vi "GUI.TestOPCConnection.vi"(8 "error in":errorcluster, 11 "Node Ptr":T1=18446744073709551615 format="%.0x") -> (0 "error out":errorcluster)   [LabVIEW 2019, in "OPC UA Client Addon System Explorer.lvlib"]
uses:
  OPC UA Client Addon System Explorer.lvlib
  <vilib>/NI VeriStand/Custom Device API/Custom Device Item Ref.ctl
  Addon Shared/SubVIs/Constants.vi
  <vilib>/NI VeriStand/Custom Device API/NI VeriStand - Get Item Property.vi
  <vilib>/NI VeriStand/Custom Device API/Get Item Property (String).vi
  <vilib>/NI VeriStand/Custom Device API/Get Item Property (U16).vi
  <vilib>/NI VeriStand/Custom Device API/Get Item Property (Dependent File).vi
  <vilib>/NI VeriStand/Custom Device API/NI VeriStand - Set Item Property.vi
  <vilib>/NI VeriStand/Custom Device API/Set Item Property (String).vi
  <vilib>/NI VeriStand/Custom Device API/Set Item Property (U16).vi
  <vilib>/Utility/libraryn.llb/Get File Extension.vi
  <vilib>/Utility/MD5Checksum.llb/MD5Checksum File.vi
  <vilib>/NI VeriStand/Custom Device API/Set Item Property (Dependent File).vi
  <vilib>/Utility/libraryn.llb/Check if File or Folder Exists.vi
  <vilib>/NI VeriStand/Custom Device API/NI VeriStand - Remove Item Property.vi
  <vilib>/OPCUA/NI OPC UA Client.lvlib
  Addon Shared/OPC UA Client Addon Shared.lvlib
  <vilib>/NI VeriStand/Custom Device API/Custom Device API.lvlib
panel:
  out "?":string="Testing..."
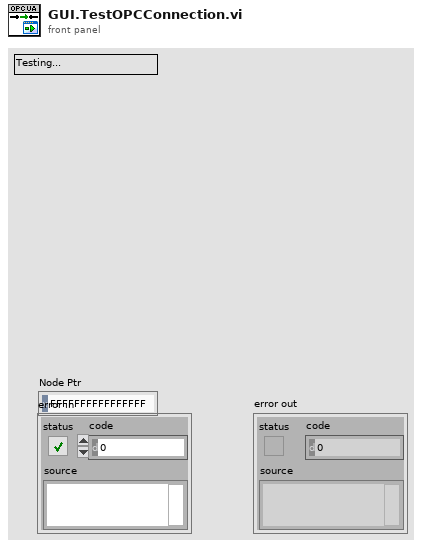
[diagram p1: front panel]
types:
  T1 = typedef "Custom Device API.lvlib/Custom Device Item Ref.ctl" = u64
  T2 = typedef "OPC UA Client Addon Shared.lvlib/OPCConnection.Properties.ctl" = cluster{"Server IP Address":string, "Server Port":u16, "Message Mode":enum16{"None", "Sign", "Sign and Encrypt"}, "Security":enum16{"Basic256", "Basic128Rsa15"}, "User Name":string, "Password":string, "Client Certificate":path, "Server Certificate":path, "Server Certificate (RT)":path, "Client Certificate (RT)":path}
  T3 = cluster{"Message Mode":enum16{"None", "Sign", "Sign and Encrypt"}, "Security":enum16{"Basic256", "Basic128Rsa15"}}
  T4 = typedef "OPC UA Client Refnum.ctl" = refnum<k21>
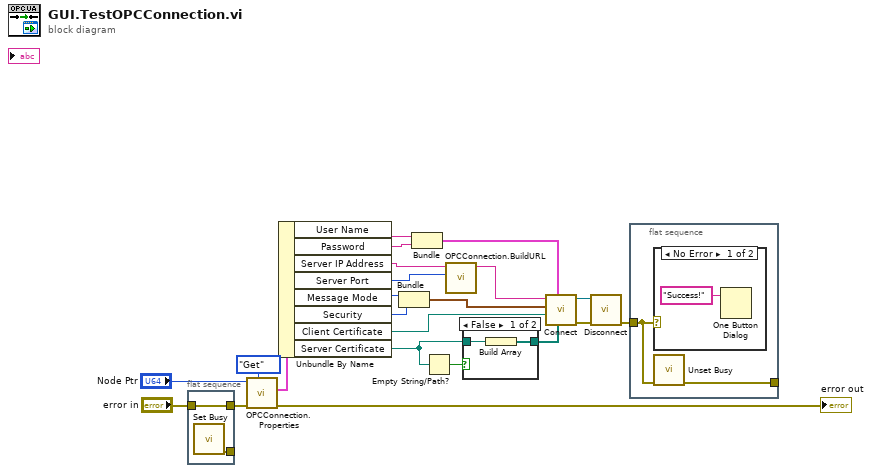
[diagram p0: block diagram]
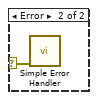
[diagram p3: hidden frame]
diagram:
  n1 = flat-sequence {
    tunnel: [w24] -> _
    tunnel: [w23] -> w5
    tunnel: "error in" -> [w23]
    frame #0 {
      n2 = call <vilib>:"Set Busy.vi"() -> ("error out"=w24:errorcluster)  [unwired: 10 in, 1 out]
    }
  }
  n3 = call "OPCConnection.Properties.vi"("Action"=enum8{"Get", "Set"}."Get", "error in (no error)"=w5, "Item Ref in"="Node Ptr") -> ("error out"=→"error out":errorcluster, "Connection.Properties"=w16:T2)  [unwired: 6 in, 1 out]
  n4 = Unbundle By Name(w16) -> ("User Name"=w9:string, "Password"=w8:string, "Server IP Address"=w15:string, "Server Port"=w14:u16, "Message Mode"=w13:enum16{"None", "Sign", "Sign and Encrypt"}, "Security"=w12:enum16{"Basic256", "Basic128Rsa15"}, "Client Certificate"=w10:path, "Server Certificate"=w1:path)
  n5 = Bundle("Message Mode"=w13, "Security"=w12) -> (w11:T3)  [unwired: 1 in]
  n6 = Bundle("User Name"=w9, "Password"=w8) -> (w7:cluster{"User Name":string, "Password":string})  [unwired: 1 in]
  n7 = Empty String/Path?(string/path=w1) -> (empty?=w2:bool)
  n8 = call "OPCConnection.BuildURL.vi"("Server Port"=w14, "Server IP Address"=w15) -> ("OPC Path"=w19:string)  [unwired: 9 in]
  n9 = case shown="False" w2 {
    tunnel: [w26 _] -> w20
    tunnel: w1 -> [w25 _]
    frame False {
      n10 = Build Array(w25) -> (w26:path[])
    }
    frame True {
    }
  }
  n11 = call <vilib>:"Connect.vi"("trusted server certificates"=w20, "username/password"=w7, "client certificate file"=w10, "security policy"=w11, "server endpoint URL"=w19) -> ("error out"=w21:errorcluster, "OPC UA client refnum out"=w22:T4)  [unwired: 4 in, 1 out]
  n12 = call <vilib>:"Disconnect.vi"("error in (no error)"=w21, "OPC UA client refnum in"=w22) -> ("error out"=w6:errorcluster)  [unwired: 9 in]
  n13 = flat-sequence {
    tunnel: w6 -> [w28]
    tunnel: [w27] -> _
    frame #0 {
      n14 = case shown="No Error" w28 {
        selector: w28 -> [_ w30]
        frame No Error {
          n15 = One Button Dialog(message="Success!") -> ()  [unwired: 1 in, 1 out]
        }
        frame Error {
          n16 = call <vilib>:"Simple Error Handler.vi"("error in (no error)"=w30) -> ()  [unwired: 4 in, 5 out]
        }
      }
      n17 = call <vilib>:"Unset Busy.vi"("error in (no error)"=w28) -> ("error out"=w27:errorcluster)  [unwired: 10 in]
    }
  }
